vi "LVClient2011.vi"() -> ()   [LabVIEW 2023]
uses:
  <vilib>/measure/NI_MABase.lvlib
panel:
  out "error out":errorcluster
  out "Waveform Chart":waveform(dbl)(graph)
  in  "error in (no error)":errorcluster
  in  "Pass":bool
  in  "Fail":bool
  in  "Stop Server":bool
  in  "Stop Client":bool
  in  "Init Button":bool
  in  "Play Button":bool
  out "TCP / IP Read (max. 9 bytes)":string
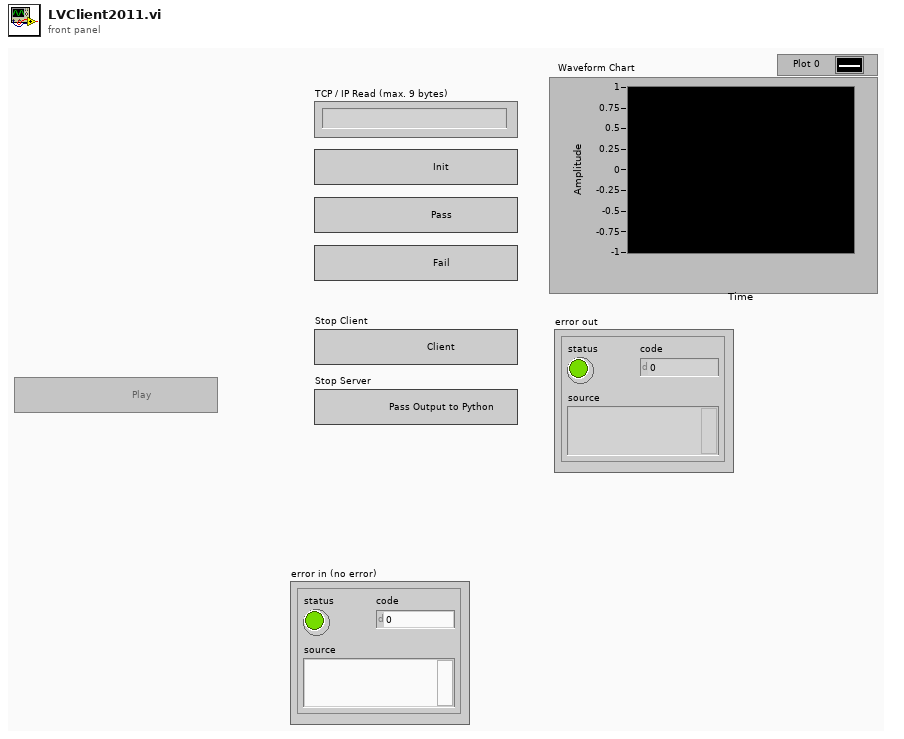
[diagram p1: front panel]
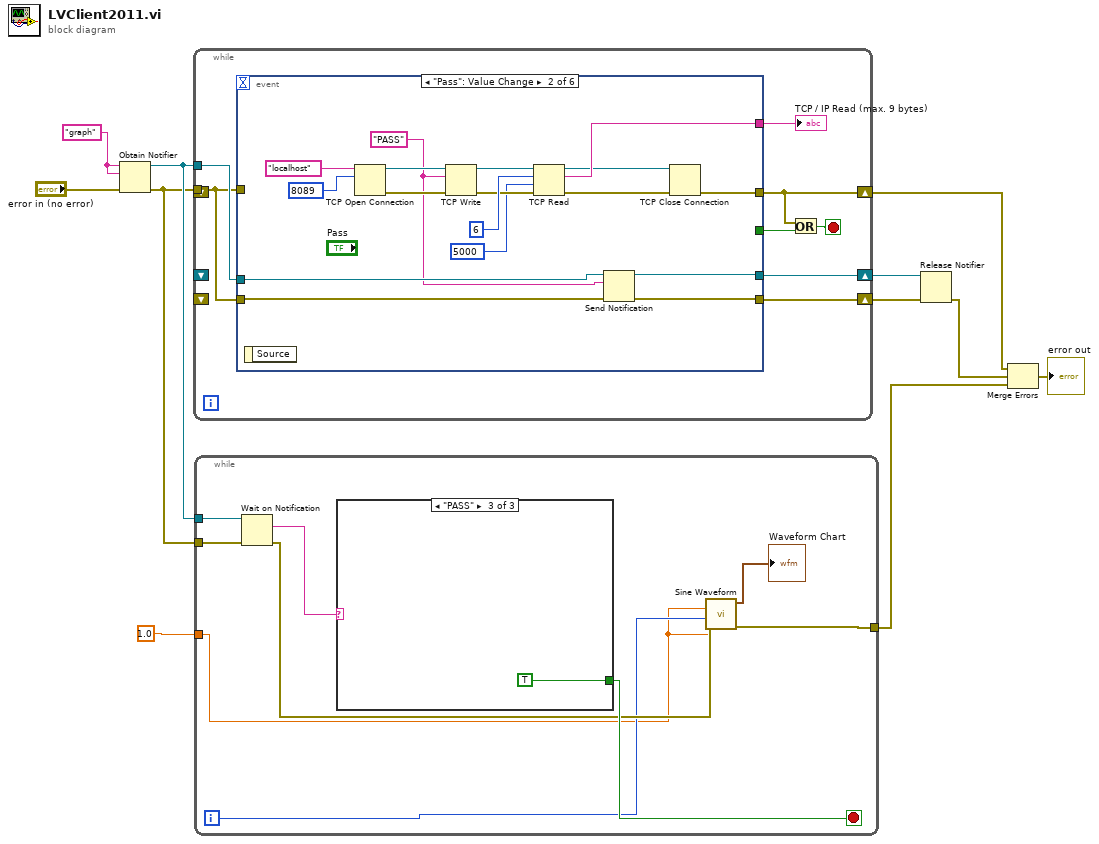
[diagram p0: block diagram]
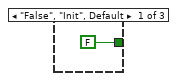
[diagram p2: hidden frame]
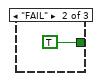
[diagram p3: hidden frame]
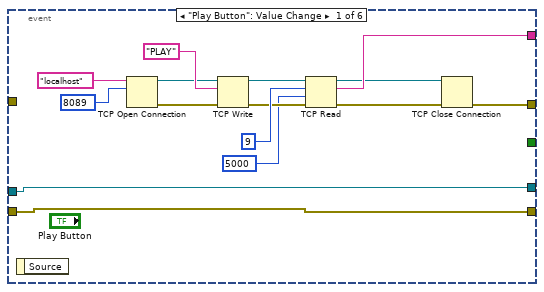
[diagram p4: hidden frame]
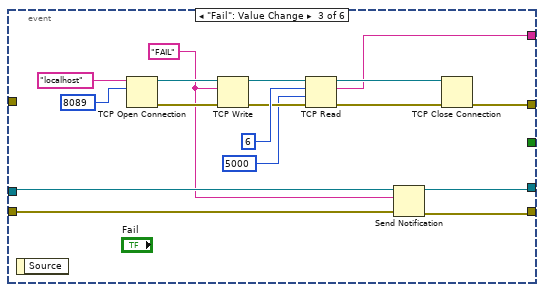
[diagram p5: hidden frame]
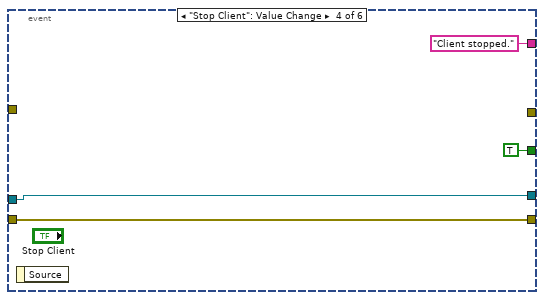
[diagram p6: hidden frame]
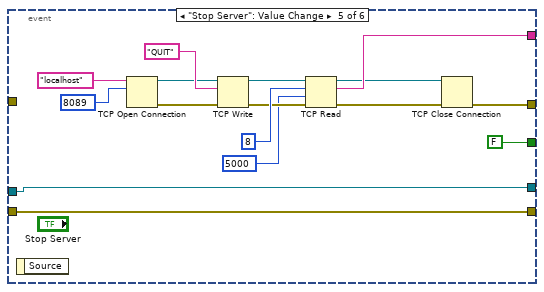
[diagram p7: hidden frame]
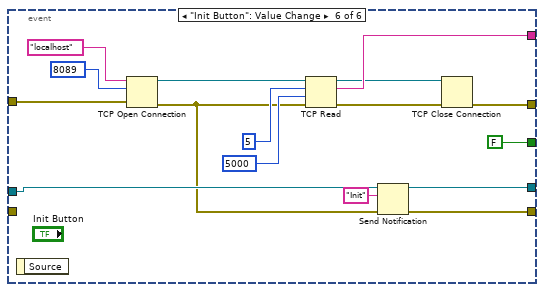
[diagram p8: hidden frame]
diagram:
  w10 = "graph" ("name (unnamed)")
  n1 = Obtain Notifier(name (unnamed)=w10, notification data type=w10, error in (no error)="error in (no error)") -> (notifier out=w9:refnum<notifier>, error out=w7:errorcluster)  [unwired: 1 in, 1 out]
  n2 = while {
    tunnel: w7 -> [w12]
    tunnel: w9 -> [w15]
    shift-right: [w18] -> w3
    shift-left: _ -> [_]
    shift-right: [w13] -> w8
    shift-left: _ -> [_]
    shift-right: [w14] -> w5
    shift-left: _ -> [_]
    stop <- w17 stop-if-true
    n3 = event shown="[1] \"Pass\": Value Change" {
      selector: _ -> [_ _ _ _ _ _]
      dyn-events: _ -> [_ _ _ _ _ _]
      timeout: _ -> [_ _ _ _ _ _]
      tunnel: [w22 w40 w58 _ w76 w97] -> w18
      tunnel: [w29 w47 w57 "Client stopped." ("data out") w83 w102] -> w19
      tunnel: [_ _ _ TRUE FALSE FALSE] -> w16
      tunnel: w12 -> [_ _ _ _ _ w94]
      tunnel: w15 -> [w21 w37 w54 w70 w74 w93]
      tunnel: [w20 w38 w55 w69 w73 w90] -> w14
      tunnel: [w21 w36 w53 w70 w74 w89] -> w13
      tunnel: w12 -> [w20 w39 w56 w69 w73 _]
      event "Play Button": Value Change {
        n4 = event-data() -> ()  [unwired: 1 in, 1 out]
        n5 = TCP Open Connection(address="localhost", remote port or service name=u16 8089) -> (connection ID=w26:refnum<k5>, error out=w25:errorcluster)  [unwired: 3 in]
        n6 = TCP Write(connection ID=w26, data in="PLAY", error in (no error)=w25) -> (connection ID out=w32:refnum<k5>, error out=w31:errorcluster)  [unwired: 1 in, 1 out]
        n7 = TCP Read(connection ID=w32, bytes to read=9, error in (no error)=w31, 9:5000 ("timeout ms (25000)")) -> (connection ID out=w24:refnum<k5>, data out=w29:string, error out=w23:errorcluster)  [unwired: 1 in]
        n8 = TCP Close Connection(connection ID=w24, error in (no error)=w23) -> (error out=w22:errorcluster)  [unwired: 1 in, 1 out]
      }
      event "Pass": Value Change {
        w35 = "PASS" ("data in")
        n9 = event-data() -> ()  [unwired: 1 in, 1 out]
        n10 = TCP Open Connection(address="localhost", remote port or service name=u16 8089) -> (connection ID=w44:refnum<k5>, error out=w43:errorcluster)  [unwired: 3 in]
        n11 = TCP Write(connection ID=w44, data in=w35, error in (no error)=w43) -> (connection ID out=w50:refnum<k5>, error out=w49:errorcluster)  [unwired: 1 in, 1 out]
        n12 = TCP Read(connection ID=w50, bytes to read=6, error in (no error)=w49, 9:5000 ("timeout ms (25000)")) -> (connection ID out=w42:refnum<k5>, data out=w47:string, error out=w41:errorcluster)  [unwired: 1 in]
        n13 = Send Notification(notification=w35, notifier=w37, error in (no error)=w39) -> (notifier out=w36:refnum<notifier>, error out=w38:errorcluster)
        n14 = TCP Close Connection(connection ID=w42, error in (no error)=w41) -> (error out=w40:errorcluster)  [unwired: 1 in, 1 out]
      }
      event "Fail": Value Change {
        w52 = "FAIL" ("data in")
        n15 = event-data() -> ()  [unwired: 1 in, 1 out]
        n16 = TCP Open Connection(address="localhost", remote port or service name=u16 8089) -> (connection ID=w62:refnum<k5>, error out=w61:errorcluster)  [unwired: 3 in]
        n17 = TCP Write(connection ID=w62, data in=w52, error in (no error)=w61) -> (connection ID out=w67:refnum<k5>, error out=w66:errorcluster)  [unwired: 1 in, 1 out]
        n18 = TCP Read(connection ID=w67, bytes to read=6, error in (no error)=w66, 9:5000 ("timeout ms (25000)")) -> (connection ID out=w60:refnum<k5>, data out=w57:string, error out=w59:errorcluster)  [unwired: 1 in]
        n19 = Send Notification(notification=w52, notifier=w54, error in (no error)=w56) -> (notifier out=w53:refnum<notifier>, error out=w55:errorcluster)
        n20 = TCP Close Connection(connection ID=w60, error in (no error)=w59) -> (error out=w58:errorcluster)  [unwired: 1 in, 1 out]
      }
      event "Stop Client": Value Change {
        n21 = event-data() -> ()  [unwired: 1 in, 1 out]
      }
      event "Stop Server": Value Change {
        n22 = event-data() -> ()  [unwired: 1 in, 1 out]
        n23 = TCP Open Connection(address="localhost", remote port or service name=u16 8089) -> (connection ID=w80:refnum<k5>, error out=w79:errorcluster)  [unwired: 3 in]
        n24 = TCP Write(connection ID=w80, data in="QUIT", error in (no error)=w79) -> (connection ID out=w86:refnum<k5>, error out=w85:errorcluster)  [unwired: 1 in, 1 out]
        n25 = TCP Read(connection ID=w86, bytes to read=8, error in (no error)=w85, 9:5000 ("timeout ms (25000)")) -> (connection ID out=w78:refnum<k5>, data out=w83:string, error out=w77:errorcluster)  [unwired: 1 in]
        n26 = TCP Close Connection(connection ID=w78, error in (no error)=w77) -> (error out=w76:errorcluster)  [unwired: 1 in, 1 out]
      }
      event "Init Button": Value Change {
        n27 = event-data() -> ()  [unwired: 1 in, 1 out]
        n28 = TCP Open Connection(address="localhost", remote port or service name=u16 8089, error in (no error)=w94) -> (connection ID=w95:refnum<k5>, error out=w92:errorcluster)  [unwired: 2 in]
        n29 = TCP Read(connection ID=w95, bytes to read=5, error in (no error)=w92, 9:5000 ("timeout ms (25000)")) -> (connection ID out=w99:refnum<k5>, data out=w102:string, error out=w98:errorcluster)  [unwired: 1 in]
        n30 = Send Notification(notification="Init" ("element"), notifier=w93, error in (no error)=w92) -> (notifier out=w89:refnum<notifier>, error out=w90:errorcluster)
        n31 = TCP Close Connection(connection ID=w99, error in (no error)=w98) -> (error out=w97:errorcluster)  [unwired: 1 in, 1 out]
      }
    }
    "TCP / IP Read (max. 9 bytes)" <- w19
    n32 = Or(x=w18, y=w16) -> (x .or. y?=w17:bool)
  }
  n33 = while {
    tunnel: w9 -> [w113]
    tunnel: w7 -> [w110]
    tunnel: [w106] -> w6
    tunnel: 1.0 ("frequency") -> [w107]
    i -> [w108]
    stop <- w111 stop-if-true
    n34 = Wait on Notification(notifier=w113, error in (no error)=w110) -> (notification=w112:string, error out=w109:errorcluster)  [unwired: 2 in, 2 out]
    n35 = case shown="\"PASS\"" w112 {
      tunnel: [FALSE TRUE TRUE] -> w111
      frame "False", "Init", Default {
      }
      frame "FAIL" {
      }
      frame "PASS" {
      }
    }
    n36 = call <vilib>:"Sine Waveform.vi"("error in (no error)"=w109, "phase"=w108, "amplitude"=w107, "frequency"=w107) -> ("error out"=w106:errorcluster, "signal out"=→"Waveform Chart":waveform(dbl))  [unwired: 6 in]
  }
  n37 = Release Notifier(notifier=w8, error in (no error)=w5) -> (error out=w4:errorcluster)  [unwired: 1 in, 2 out]
  n38 = Merge Errors(w3, w4, w6) -> (→"error out":errorcluster)
